vi "服务器2.vi"() -> ()   [LabVIEW 2020]
uses:
  <vilib>/Analysis/NI_AALBase.lvlib
panel:
  out "错误输出":errorcluster
  in  "port":u16 caption="端口"
  in  "停止":bool
  out "波形图表":dbl[](graph)
  in  "cycles":dbl=1.0 caption="周期" format="%0.2f"
  in  "phase(degrees)":dbl caption="相位（度）" format="%0.2f"
  in  "amplitude":dbl=1.0 caption="幅值" format="%0.2f"
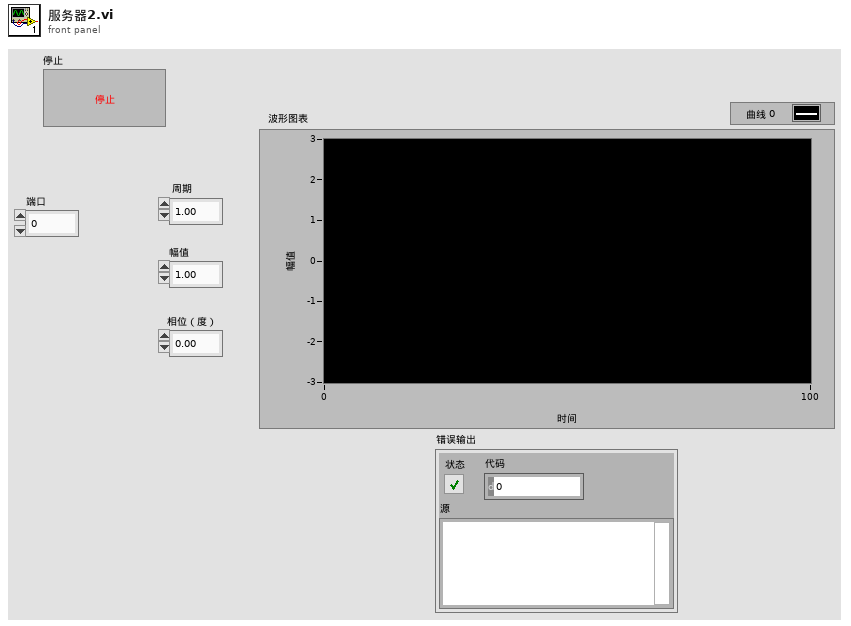
[diagram p1: front panel]
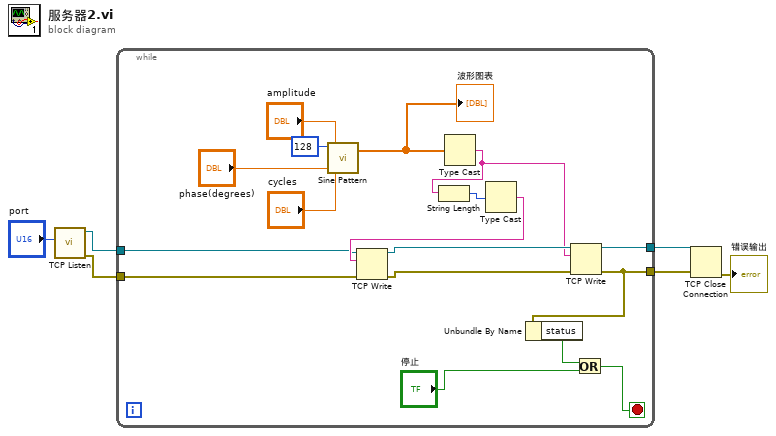
[diagram p0: block diagram]
diagram:
  n1 = call <vilib>:"TCP Listen.vi"("port"="port") -> ("error out"=w4:errorcluster, "connection ID"=w3:refnum<k5>)  [unwired: 6 in, 3 out]
  n2 = while {
    tunnel: [w22] -> w6
    tunnel: [w10] -> w5
    tunnel: w4 -> [w12]
    tunnel: w3 -> [w11]
    stop <- w8 stop-if-true
    n3 = call <vilib>:"Sine Pattern.vi"("cycles"="cycles", "phase(degrees)"="phase(degrees)", "amplitude"="amplitude", "samples"=128) -> ("Sinusoidal Pattern"=w17:dbl[])  [unwired: 1 out]
    "波形图表" <- w17
    n4 = Type Cast(x=w17) -> (*(type *) &x=w14:string)  [unwired: 1 in]
    n5 = String Length(string=w14) -> (length=w16:i32)
    n6 = Type Cast(x=w16) -> (*(type *) &x=w15:string)  [unwired: 1 in]
    n7 = TCP Write(connection ID=w11, data in=w15, error in (no error)=w12) -> (connection ID out=w23:refnum<k5>, error out=w13:errorcluster)  [unwired: 1 in, 1 out]
    n8 = TCP Write(connection ID=w23, data in=w14, error in (no error)=w13) -> (connection ID out=w22:refnum<k5>, error out=w10:errorcluster)  [unwired: 1 in, 1 out]
    n9 = Unbundle By Name(w10) -> ("status"=w9:bool)
    n10 = Or(x=w9, y="停止") -> (x .or. y?=w8:bool)
  }
  n11 = TCP Close Connection(connection ID=w6, error in (no error)=w5) -> (error out=→"错误输出":errorcluster)  [unwired: 1 in, 1 out]
